vi "Read.vi"(5 "Keep Bus Busy":bool, 6 "Timeout ms (1000)":i32=1000, 7 "error in (no error)":errorcluster, 8 "Byte Count":u32, 9 "Slave Address (7-bit)":u8, 10 "I2C Ref In":T1={"myRIO Reference"={"myRIO Model"=enum."Unknown", "myRIO Hardware Reference"={"Generic FPGA Reference"=refnum, "Allow multiple opens"=FALSE}}, "I2C Channels Enum"=enum."Not Connected", "I2C Configuration"={"I2C Transfer Rate"=enum."Fast mode (400 kbps)"}}) -> (0 "error out":errorcluster, 2 "Bytes Read":u8[](array[numeric]), 3 "I2C Ref Out":T1={"myRIO Reference"={"myRIO Model"=enum."Unknown", "myRIO Hardware Reference"={"Generic FPGA Reference"=refnum, "Allow multiple opens"=FALSE}}, "I2C Channels Enum"=enum."Not Connected", "I2C Configuration"={"I2C Transfer Rate"=enum."Fast mode (400 kbps)"}})   [LabVIEW 2021, in "I2C.lvlib"]
doc: "Reads a specified number of bytes of data from an Inter-Integrated Circuit (I2C) channel. This VI returns the result when finishing reading all the bytes or when timing out."
uses:
  <vilib>/myRIO/Instrument Drivers/Onboard IO/I2C/I2C.lvlib
  <vilib>/myRIO/Instrument Drivers/Onboard IO/I2C/typedefs/I2C Reference.ctl
  <vilib>/myRIO/Common/Instrument Driver Framework/Utilities/typedefs/myRIO Generic Hardware Reference.ctl
  <vilib>/myRIO/Common/Instrument Driver Framework/Utilities/typedefs/Hardware Version Enum.ctl
  <vilib>/myRIO/Common/Instrument Driver Framework/Utilities/typedefs/myRIO v1.0 Reference.ctl
  <vilib>/myRIO/Common/Instrument Driver Framework/Utilities/typedefs/Generic FPGA Reference.ctl
  <vilib>/myRIO/Common/Instrument Driver Framework/myRIO v1.0/I2C/typedefs/I2C Channels Enum.ctl
  <vilib>/myRIO/Instrument Drivers/Onboard IO/I2C/typedefs/I2C Configuration.ctl
  <vilib>/myRIO/Instrument Drivers/Onboard IO/I2C/typedefs/I2C Transfer Rate.ctl
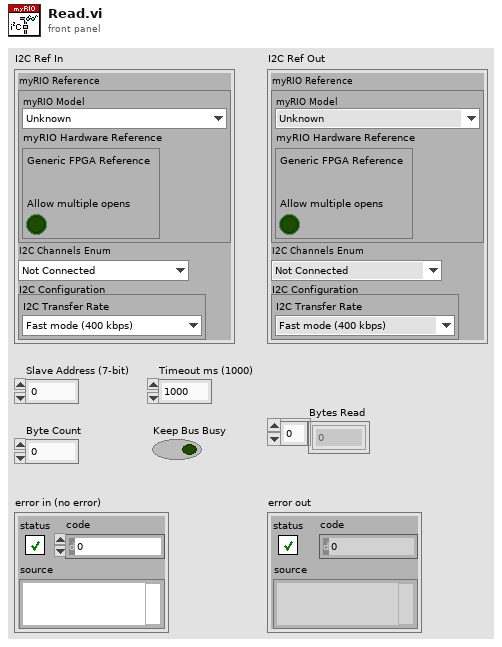
[diagram p1: front panel]
types:
  T1 = typedef "I2C.lvlib/I2C Reference.ctl" = cluster{"myRIO Reference":T2, "I2C Channels Enum":T6, "I2C Configuration":T7}
  T2 = typedef "myRIO Generic Hardware Reference.ctl" = cluster{"myRIO Model":T3, "myRIO Hardware Reference":T4}
  T3 = typedef "Hardware Version Enum.ctl" = enum16{"Unknown", "myRIO-1900", "myRIO-1950", "roboRIO", "NI ELVIS RIO CM", "ELVIS III"}
  T4 = typedef "myRIO v1.0 Reference.ctl" = cluster{"Generic FPGA Reference":T5, "Allow multiple opens":bool}
  T5 = typedef "Generic FPGA Reference.ctl" = refnum<k20>
  T6 = typedef "I2C Channels Enum.ctl" = enum16{"Not Connected", "A/I2C", "B/I2C", "I2C/I2C"}
  T7 = typedef "I2C.lvlib/I2C Configuration.ctl" = cluster{"I2C Transfer Rate":T8}
  T8 = typedef "I2C.lvlib/I2C Transfer Rate.ctl" = enum16{"Standard mode (100 kbps)", "Fast mode (400 kbps)"}
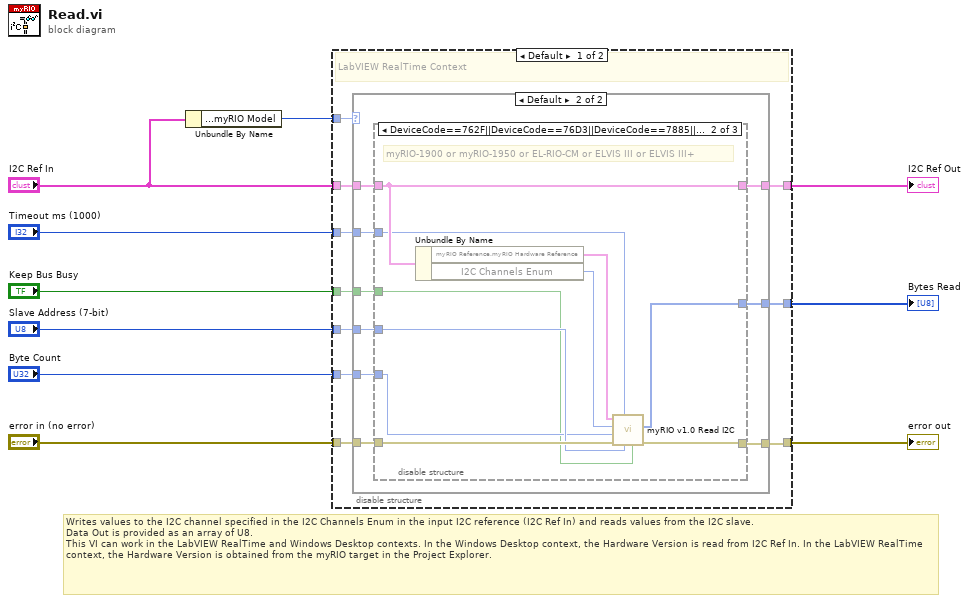
[diagram p0: block diagram]
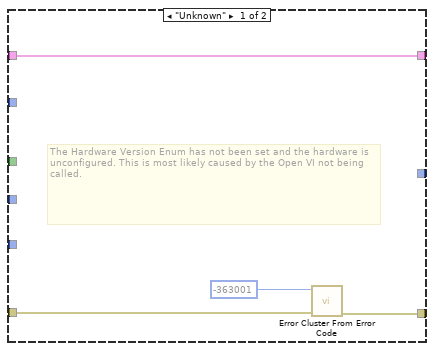
[diagram p2: hidden frame]
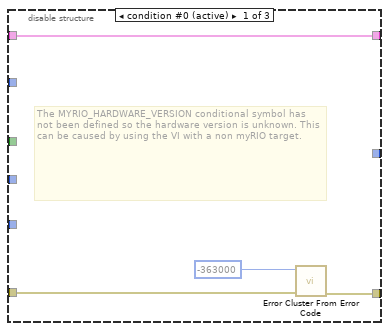
[diagram p3: hidden frame]
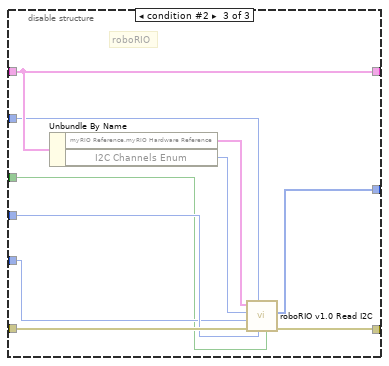
[diagram p4: hidden frame]
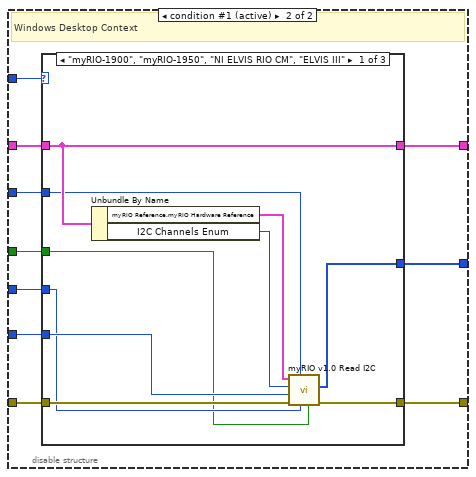
[diagram p5: hidden frame]
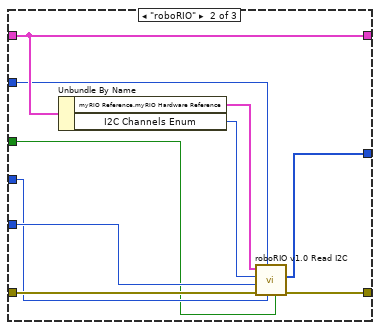
[diagram p6: hidden frame]
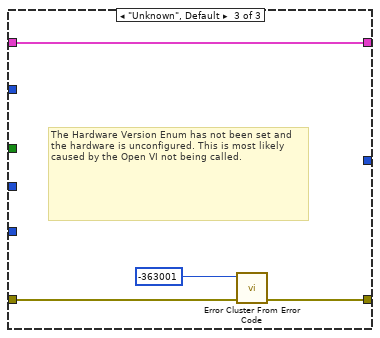
[diagram p7: hidden frame]
diagram:
  # "Writes values to the I2C channel specified in the I2C Channels Enum in the input I2C reference (I2C Ref In) and reads values from the I2C slave.\nData Out is provided as an array of U8.\nThis VI can work in the LabVIEW RealTime and Windows Desktop contexts. In the Windows Desktop context, the Hardware Version is read from I2C Ref In. In the LabVIEW RealTime context, the Hardware Version is obtained from the myRIO target in the Project Explorer."
  n1 = Unbundle By Name("I2C Ref In") -> ("myRIO Reference.myRIO Model"=w3:T3)
  n2 = disable-structure shown="Default" {
    disable-tunnel: [w20 w67] -> w7
    disable-tunnel: "I2C Ref In" -> [w19 w64]
    disable-tunnel: "error in (no error)" -> [w18 w66]
    disable-tunnel: [w17 w65] -> w8
    disable-tunnel: w3 -> [w16 w63]
    disable-tunnel: [w15 w62] -> w6
    disable-tunnel: "Byte Count" -> [w13 w61]
    disable-tunnel: "Slave Address (7-bit)" -> [w14 w60]
    disable-tunnel: "Keep Bus Busy" -> [w12 w59]
    disable-tunnel: "Timeout ms (1000)" -> [w11 w58]
    frame condition #0 {
      # "LabVIEW RealTime Context"
      n3 = case shown="Default" w16 {
        tunnel: [w23 w33] -> w20
        tunnel: w19 -> [w21 w32]
        tunnel: w18 -> [w22 w31]
        tunnel: [w21 w30] -> w17
        tunnel: [_ w29] -> w15
        tunnel: w14 -> [_ w28]
        tunnel: w13 -> [_ w27]
        tunnel: w12 -> [_ w26]
        tunnel: w11 -> [_ w25]
        frame "Unknown" {
          # "The Hardware Version Enum has not been set and the hardware is unconfigured. This is most likely caused by the Open VI not being called."
          n4 = call <vilib>:"Error Cluster From Error Code.vi"("error in (no error)"=w22, "error code (0)"=-363001) -> ("error out"=w23:errorcluster)  [unwired: 7 in]
        }
        frame Default {
          n5 = disable-structure shown="DeviceCode==762F||DeviceCode==76D3||DeviceCode==7885||DeviceCode==7928||DeviceCode==793C" {
            disable-tunnel: w32 -> [w34 w45 w55]
            disable-tunnel: [w37 w43 w53] -> w33
            disable-tunnel: w31 -> [w35 w44 w54]
            disable-tunnel: [w34 w45 w55] -> w30
            disable-tunnel: [_ w42 w52] -> w29
            disable-tunnel: w28 -> [_ w41 w51]
            disable-tunnel: w27 -> [_ w40 w50]
            disable-tunnel: w26 -> [_ w39 w49]
            disable-tunnel: w25 -> [_ w38 w48]
            frame condition #0 (active) {
              # "The MYRIO_HARDWARE_VERSION conditional symbol has not been defined so the hardware version is unknown. This can be caused by using the VI with a non myRIO target."
              n6 = call <vilib>:"Error Cluster From Error Code.vi"("error in (no error)"=w35, "error code (0)"=-363000) -> ("error out"=w37:errorcluster)  [unwired: 7 in]
            }
            frame condition #1 {
              # "myRIO-1900 or myRIO-1950 or EL-RIO-CM or ELVIS III or ELVIS III+"
              n7 = Unbundle By Name(w45) -> ("myRIO Reference.myRIO Hardware Reference"=w47:T4, "I2C Channels Enum"=w46:T6)
              n8 = call <vilib>:"myRIO v1.0 Read I2C.vi"("Keep Bus Busy"=w39, "Slave Address (7-bit)"=w41, "Timeout ms (1000)"=w38, "Error In (No Error)"=w44, "Bytes to Read"=w40, "Channel"=w46, "myRIO Ref In"=w47) -> ("error out"=w43:errorcluster, "Data Read"=w42:u8[])  [unwired: 2 in, 1 out]
            }
            frame condition #2 {
              # "roboRIO"
              n9 = Unbundle By Name(w55) -> ("myRIO Reference.myRIO Hardware Reference"=w57:T4, "I2C Channels Enum"=w56:T6)
              n10 = call <vilib>:"roboRIO v1.0 Read I2C.vi"("Keep Bus Busy"=w49, "Slave Address (7-bit)"=w51, "Timeout ms (1000)"=w48, "Error In (No Error)"=w54, "Bytes to Read"=w50, "Channel"=w56, "myRIO Ref In"=w57) -> ("error out"=w53:errorcluster, "Data Read"=w52:u8[])  [unwired: 2 in, 1 out]
            }
          }
        }
      }
    }
    frame condition #1 (active) {
      # "Windows Desktop Context"
      n11 = case shown="\"myRIO-1900\", \"myRIO-1950\", \"NI ELVIS RIO CM\", \"ELVIS III\"" w63 {
        tunnel: [w74 w84 w91] -> w67
        tunnel: w64 -> [w75 w85 w88]
        tunnel: w66 -> [w73 w83 w89]
        tunnel: [w75 w85 w88] -> w65
        tunnel: [w72 w82 _] -> w62
        tunnel: w61 -> [w71 w81 _]
        tunnel: w60 -> [w70 w80 _]
        tunnel: w59 -> [w69 w79 _]
        tunnel: w58 -> [w68 w78 _]
        frame "myRIO-1900", "myRIO-1950", "NI ELVIS RIO CM", "ELVIS III" {
          n12 = Unbundle By Name(w75) -> ("myRIO Reference.myRIO Hardware Reference"=w77:T4, "I2C Channels Enum"=w76:T6)
          n13 = call <vilib>:"myRIO v1.0 Read I2C.vi"("Keep Bus Busy"=w69, "Slave Address (7-bit)"=w70, "Timeout ms (1000)"=w68, "Error In (No Error)"=w73, "Bytes to Read"=w71, "Channel"=w76, "myRIO Ref In"=w77) -> ("error out"=w74:errorcluster, "Data Read"=w72:u8[])  [unwired: 2 in, 1 out]
        }
        frame "roboRIO" {
          n14 = Unbundle By Name(w85) -> ("myRIO Reference.myRIO Hardware Reference"=w87:T4, "I2C Channels Enum"=w86:T6)
          n15 = call <vilib>:"roboRIO v1.0 Read I2C.vi"("Keep Bus Busy"=w79, "Slave Address (7-bit)"=w80, "Timeout ms (1000)"=w78, "Error In (No Error)"=w83, "Bytes to Read"=w81, "Channel"=w86, "myRIO Ref In"=w87) -> ("error out"=w84:errorcluster, "Data Read"=w82:u8[])  [unwired: 2 in, 1 out]
        }
        frame "Unknown", Default {
          # "The Hardware Version Enum has not been set and the hardware is unconfigured. This is most likely caused by the Open VI not being called."
          n16 = call <vilib>:"Error Cluster From Error Code.vi"("error in (no error)"=w89, "error code (0)"=-363001) -> ("error out"=w91:errorcluster)  [unwired: 7 in]
        }
      }
    }
  }
  "I2C Ref Out" <- w8
  "error out" <- w7
  "Bytes Read" <- w6
